vi "Test Norm Dist.vi"() -> ()   [LabVIEW 2020, in "Tone Cloud.lvclass"]
uses:
  Tone Cloud.lvclass
  Serialized.ctl
  Spacing.ctl
  Level Mode.ctl
  Tone Cloud.lvclass/Tone Cloud.ctl
  Utility VIs/Math VIs/LinSpace (x0-dx-npts).vi
  <vilib>/Analysis/NI_AALPro.lvlib
panel:
  out "Histogram":T1(graph)={"X Values"=[0.0, 1.0, 2.0, 3.0, 4.0, 5.0, 6.0, 7.0, 8.0, 9.0, 10.0, 11.0, 12.0, 13.0, 14.0, 15.0, 16.0, 17.0, 18.0, 19.0, 20.0, 21.0, 22.0, 23.0, 24.0, 25.0, 26.0, 27.0, 28.0, 29.0, 30.0, 31.0, 32.0, 33.0, 34.0, 35.0, 36.0, 37.0, 38.0, 39.0, 40.0, 41.0, 42.0, 43.0, 44.0, 45.0, 46.0, 47.0, 48.0], "Histogram: h(x)"=[0, 0, 0, 1, 1, 1, 9, 18, 20, 78, 112, 215, 330, 578, 870, 1292, 1886, 2693, 3422, 4289, 5419, 6099, 6984, 7639, 7952, 7934, 7567, 6919, 6217, 5441, 4406, 3545, 2476, 1861, 1384, 938, 586, 355, 208, 111, 71, 42, 20, 5, 3, 0, 2, 0, 1]}
  in  "Nclock":i32=1000
  in  "Fs (Hz)":dbl=100000.0
  in  "Std Dev":dbl
  in  "Mean":dbl
  in  "Serialized":T2
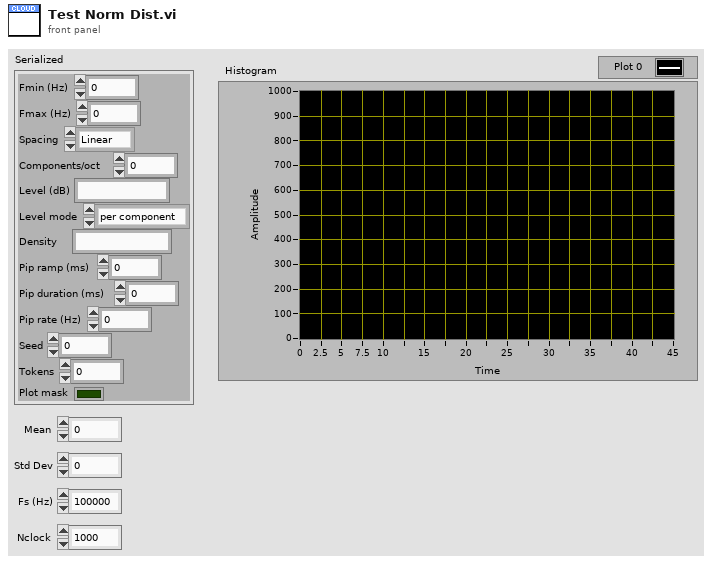
[diagram p1: front panel]
types:
  T1 = cluster{"X Values":dbl[], "Histogram: h(x)":i32[]}
  T2 = typedef "Tone Cloud.lvclass/Serialized.ctl" = cluster{"Fmin (Hz)":dbl, "Fmax (Hz)":dbl, "Spacing":T3, "Components/oct":dbl, "Level (dB)":string, "Level mode":T4, "Density":string, "Pip ramp (ms)":dbl, "Pip duration (ms)":dbl, "Pip rate (Hz)":dbl, "Seed":i32, "Tokens":i32, "Plot mask":bool}
  T3 = typedef "Tone Cloud.lvclass/Spacing.ctl" = enum16{"Linear", "Log"}
  T4 = typedef "Tone Cloud.lvclass/Level Mode.ctl" = enum16{"per component", "total rms"}
  T5 = cluster{dbl, dbl, "inclusion":enum32{"lower", "upper"}}
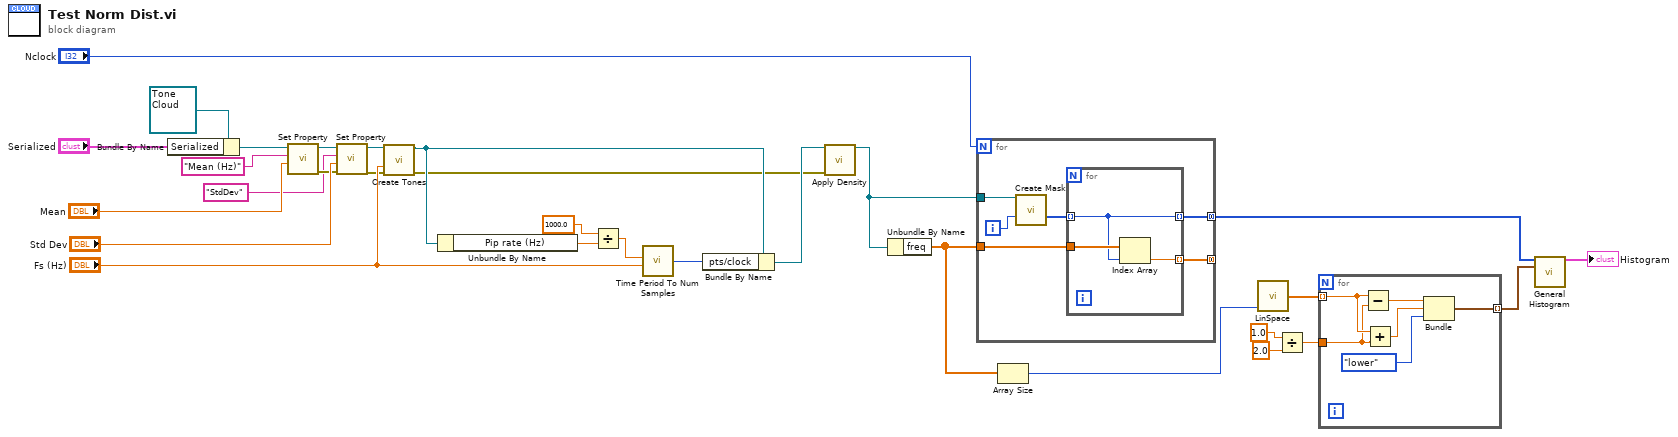
[diagram p0: block diagram]
diagram:
  n1 = Bundle By Name(cluster=refnum<class "Tone Cloud.lvclass"> refnum ("ToneCloud in"), "Serialized"="Serialized") -> (w10:refnum<class "Tone Cloud.lvclass">)
  n2 = call-dynamic "Set Property.vi"("Value"="Mean", "Property"="Mean (Hz)", "ToneCloud in"=w10) -> ("error out"=w2:errorcluster, "ToneCloud out"=w7:refnum<class "Tone Cloud.lvclass">)  [unwired: 7 in]
  n3 = call-dynamic "Set Property.vi"("error in (no error)"=w2, "Value"="Std Dev", "Property"="StdDev", "ToneCloud in"=w7) -> ("error out"=w5:errorcluster, "ToneCloud out"=w6:refnum<class "Tone Cloud.lvclass">)  [unwired: 6 in]
  n4 = call "Create Tones.vi"("ToneCloud in"=w6, "Fs (Hz)"="Fs (Hz)", "error in (no error)"=w5) -> ("ToneCloud out"=w29:refnum<class "Tone Cloud.lvclass">, "error out"=w4:errorcluster)  [unwired: 11 in]
  n5 = Unbundle By Name(w29) -> ("Pip rate (Hz)"=w25:dbl)
  n6 = Divide(x=1000.0, y=w25) -> (x/y=w27:dbl)
  n7 = call "Time Period To Num Samples.vi"("Duration (ms)"=w27, "Sampling rate (Hz)"="Fs (Hz)") -> ("Samples"=w28:i32)  [unwired: 5 in]
  n8 = Bundle By Name(cluster=w29, "pts/clock"=w28) -> (w30:refnum<class "Tone Cloud.lvclass">)
  n9 = call "Apply Density.vi"("ToneCloud in"=w30, "error in (no error)"=w4) -> ("ToneCloud out"=w22:refnum<class "Tone Cloud.lvclass">)  [unwired: 12 in, 1 out]
  n10 = Unbundle By Name(w22) -> ("freq"=w14:dbl[])
  n11 = for {
    N: "Nclock" -> [_]
    tunnel: w14 -> [w36]
    tunnel: w22 -> [w35]
    tunnel: [w32] -> _ mode=concatenating
    tunnel: [w31] -> w16 mode=concatenating
    i -> [w34]
    n12 = call "Create Mask.vi"("ToneCloud in"=w35, "iRow"=w34) -> ("indices"=w33:i32[])  [unwired: 9 in, 4 out]
    n13 = for {
      tunnel: w36 -> [w39]
      tunnel: w33 -> [w37] mode=indexing
      tunnel: [w38] -> w32 mode=indexing
      tunnel: [w37] -> w31 mode=indexing
      n14 = Index Array(array=w39, index=w37) -> (element=w38:dbl)
    }
  }
  n15 = Array Size(array=w14) -> (size(s)=w13:i32)
  n16 = call-poly "LinSpace.vi"("npts"=w13) -> ("Array"=w15:dbl[])  [unwired: 3 in, 1 out]
  n17 = Divide(x=1.0, y=2.0) -> (x/y=w19:dbl)
  n18 = for {
    tunnel: w15 -> [w45] mode=indexing
    tunnel: w19 -> [w44]
    tunnel: [w40] -> w18 mode=indexing
    n19 = Subtract(x=w45, y=w44) -> (x-y=w43:dbl)
    n20 = Add(x=w45, y=w44) -> (x+y=w42:dbl)
    n21 = Bundle(w43, w42, "inclusion"=enum32{"lower", "upper"}."lower") -> (w40:T5)  [unwired: 1 in]
  }
  n22 = call <vilib>:"General Histogram.vi"("X"=w16, "Bins"=w18) -> ("Histogram Graph"=→"Histogram":T1)  [unwired: 9 in, 4 out]
